vi "Delete Unused Pictures.vi"(8 "error in (no error)":errorcluster, 9 "Current Pictures Paths In":path[](array[path]), 11 "Pictures Folder In":path) -> (0 "error out":errorcluster)   [LabVIEW 2011]
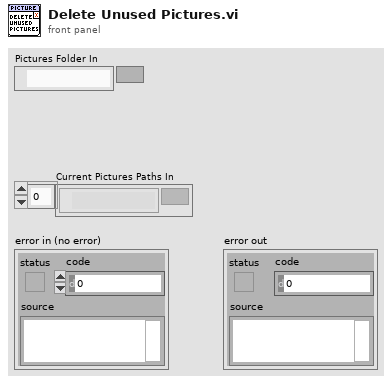
[diagram p1: front panel]
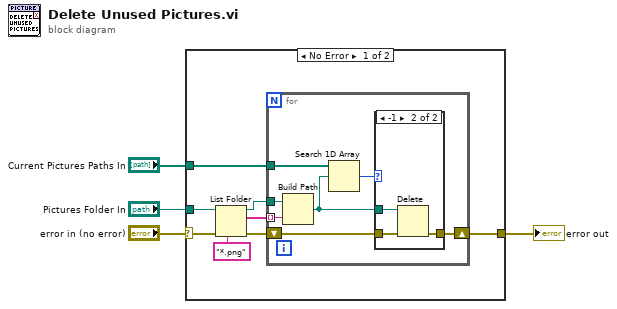
[diagram p0: block diagram]
diagram:
  n1 = case shown="No Error" "error in (no error)" {
    selector: "error in (no error)" -> [w7 w24]
    tunnel: [w12 w24] -> w4
    tunnel: "Current Pictures Paths In" -> [w11 _]
    tunnel: "Pictures Folder In" -> [w9 _]
    frame No Error {
      n2 = List Folder(path=w9, pattern="*.png", error in=w7) -> (path out=w8:path, filenames=w5:string[], error out=w6:errorcluster)  [unwired: 1 in, 1 out]
      n3 = for {
        tunnel: w5 -> [w19] mode=indexing
        tunnel: w8 -> [w18]
        tunnel: w11 -> [w17]
        shift-right: [w14] -> w12
        shift-left: w6 -> [w13]
        n4 = Build Path(base path=w18, name or relative path=w19) -> (appended path=w15:path)
        n5 = Search 1D Array(1D array=w17, element=w15) -> (index of element=w16:i32)  [unwired: 1 in]
        n6 = case shown="-1" w16 {
          tunnel: w15 -> [_ w23]
          tunnel: [w20 w22] -> w14
          tunnel: w13 -> [w20 w21]
          frame Default {
          }
          frame -1 {
            n7 = Delete(path (use dialog)=w23, error in=w21) -> (error out=w22:errorcluster)  [unwired: 3 in, 2 out]
          }
        }
      }
    }
    frame Error {
    }
  }
  "error out" <- w4
